vi "Finish.vi"   [LabVIEW 2016]
doc: "This VI is called just before exiting. It is expected to close I/O refnum, save collected data, etc."
uses:
  <vilib>/Rock Robotics/WPI/Utilities/WPI_GetSetVariantRefNum.vi
types:
  T1 = typedef "WPI_MotorControlDeviceRef.ctl" = cluster{"DeviceStatus":errorcluster, "Type":T2, "PWM":cluster{"PWM Channel":T3, "DeadBand":T4}, "CAN":cluster{"Device Number":u8, "SetOutput VI Ref":variant, "GetOutput VI Ref":variant, "Enable VI Ref":variant, "Disable VI Ref":variant, "Data":variant}, "Invert":bool}
  T2 = typedef "WPI_MotorControlType.ctl" = enum16{"PWM", "CAN"}
  T3 = typedef "FPGA_DIOPWMChannel.ctl" = enum8{"PWM 0", "PWM 1", "PWM 2", "PWM 3", "PWM 4", "PWM 5", "PWM 6", "PWM 7", "PWM 8", "PWM 9", "PWM MXP 0", "PWM MXP 1", "PWM MXP 2", "PWM MXP 3", "PWM MXP 4", "PWM MXP 5", "PWM MXP 6", "PWM MXP 7", "PWM MXP 8", "PWM MXP 9", "Invalid"}
  T4 = typedef "WPI_PWMDeadband.ctl" = cluster{"Name":string, "maxPositivePwm":i32, "minPositivePwm":i32, "centerPwm":i32, "maxNegativePwm":i32, "minNegativePwm":i32, "angularRange":u16}
  T5 = typedef "WPI_JoystickDevRef.ctl" = cluster{"Device":T6}
  T6 = typedef "WPI_JoystickDeviceEnum.ctl" = enum16{"USB 0", "USB 1", "USB 2", "USB 3", "USB 4", "USB 5"}
  T7 = typedef "WPI_SolenoidDevRef.ctl" = cluster{"DevStatus":errorcluster, "Pneumatics Control Module":u8, "Forward Solenoid Channel":T8, "Reverse Solenoid Channel":T8}
  T8 = typedef "WPI_SolenoidChannel.ctl" = enum8{"Solenoid 0", "Solenoid 1", "Solenoid 2", "Solenoid 3", "Solenoid 4", "Solenoid 5", "Solenoid 6", "Solenoid 7", "Invalid"}
  T9 = typedef "WPI_CompressorDevRef.ctl" = cluster{"DevStatus":errorcluster, "Pneumatics Control Module":u8}
  T10 = typedef "WPI_EncoderDevRef.ctl" = cluster{"DevStatus":errorcluster, "EncoderIndex":T11, "CounterIndex":T12, "DistancePerCount":dbl, "Decoding Type":T13}
  T11 = typedef "FPGA_EncoderIdx.ctl" = enum8{"Enc 0", "Enc 1", "Enc 2", "Enc 3", "Enc 4", "Enc 5", "Enc 6", "Enc 7", "Invalid"}
  T12 = typedef "FPGA_CounterCtrSystemIndex.ctl" = enum8{"Ctr 0", "Ctr 1", "Ctr 2", "Ctr 3", "Ctr 4", "Ctr 5", "Ctr 6", "Ctr 7", "Invalid"}
  T13 = typedef "WPI_EncoderType.ctl" = enum16{"1x", "2x", "4x"}
  T14 = typedef "WPI_GyroDevRef.ctl" = cluster{"DevStatus":errorcluster, "Analog Channel":T15, "Offset":dbl, "Gain (VoltsPerDegree/Second)":dbl, "Gyro Type":enum16{"Analog", "XRS450"}, "Handle":i32, "SPI Bus":T16, "Device Found":bool, "Sample Rate":dbl, "Calibrate On Open":bool}
  T15 = typedef "FPGA_AIChannel.ctl" = enum8{"AI 0", "AI 1", "AI 2", "AI 3", "AI MXP 0", "AI MXP 1", "AI MXP 2", "AI MXP 3", "Invalid"}
  T16 = typedef "spi_bus.ctl" = enum16{"SPI On-Board, CS0", "SPI On-Board, CS1", "SPI On-Board, CS2", "SPI On-Board, CS3", "SPI MXP", "Invalid"}
  T17 = typedef "WPI_RobotDriveDevRef.ctl" = cluster{"DevStatus":errorcluster, "Motors[]":T1[], "Square Inputs":bool, "Max Output":dbl}
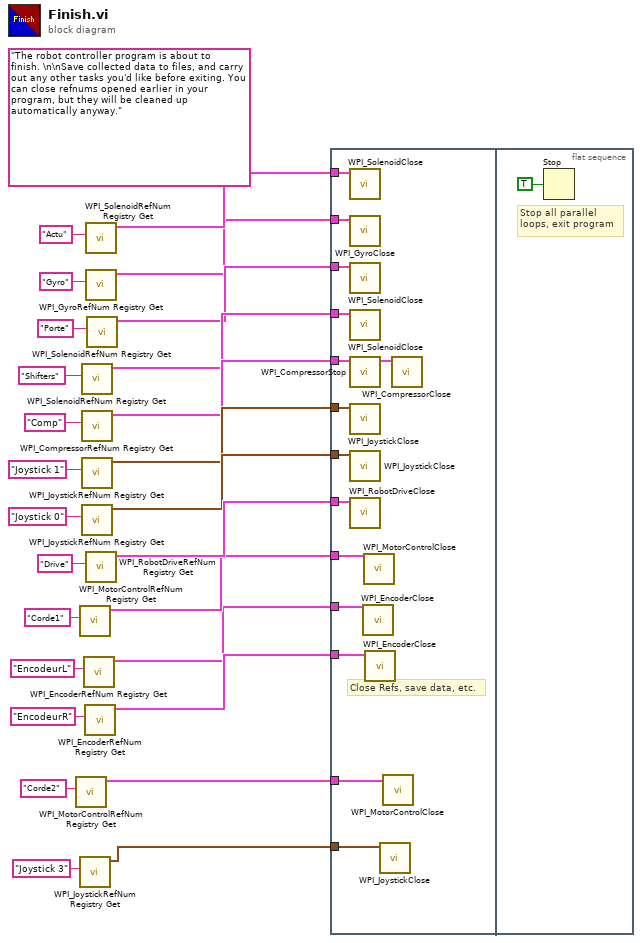
[diagram p0: block diagram]
diagram:
  (unwired) "The robot controller program is about to finish. \n\nSave collected data to files, and carry out any other tasks you'd like before exiting. You can close refnums opened earlier in your program, but they will be cleaned up automatically anyway."
  n1 = call <vilib>:"WPI_MotorControlRefNum Registry Get.vi"("refnum name"="Corde2") -> ("MotorControlDevRef"=w3:T1)  [unwired: 9 in, 1 out]
  n2 = call <vilib>:"WPI_MotorControlRefNum Registry Get.vi"("refnum name"="Corde1") -> ("MotorControlDevRef"=w10:T1)  [unwired: 9 in, 1 out]
  n3 = call <vilib>:"WPI_JoystickRefNum Registry Get.vi"("refnum name"="Joystick 3") -> ("JoystickDevRef"=w4:T5)  [unwired: 9 in, 1 out]
  n4 = call <vilib>:"WPI_SolenoidRefNum Registry Get.vi"("refnum name"="Shifters") -> ("SolenoidDevRef"=w18:T7)  [unwired: 9 in, 1 out]
  n5 = call <vilib>:"WPI_CompressorRefNum Registry Get.vi"("refnum name"="Comp") -> ("CompressorDevRef"=w20:T9)  [unwired: 9 in, 1 out]
  n6 = call <vilib>:"WPI_JoystickRefNum Registry Get.vi"("refnum name"="Joystick 1") -> ("JoystickDevRef"=w21:T5)  [unwired: 1 in, 9 out]
  n7 = call <vilib>:"WPI_JoystickRefNum Registry Get.vi"("refnum name"="Joystick 0") -> ("JoystickDevRef"=w23:T5)  [unwired: 1 in, 9 out]
  n8 = call <vilib>:"WPI_EncoderRefNum Registry Get.vi"("refnum name"="EncodeurL") -> ("EncoderDevRef"=w6:T10)  [unwired: 9 in, 1 out]
  n9 = call <vilib>:"WPI_EncoderRefNum Registry Get.vi"("refnum name"="EncodeurR") -> ("EncoderDevRef"=w8:T10)  [unwired: 9 in, 1 out]
  n10 = call <vilib>:"WPI_SolenoidRefNum Registry Get.vi"("refnum name"="Actu") -> ("SolenoidDevRef"=w16:T7)  [unwired: 9 in, 1 out]
  n11 = call <vilib>:"WPI_GyroRefNum Registry Get.vi"("refnum name"="Gyro") -> ("GyroDevRef"=w12:T14)  [unwired: 9 in, 1 out]
  n12 = call <vilib>:"WPI_RobotDriveRefNum Registry Get.vi"("refnum name"="Drive") -> ("RobotDriveDevRef"=w24:T17)  [unwired: 1 in, 9 out]
  n13 = call <vilib>:"WPI_SolenoidRefNum Registry Get.vi"("refnum name"="Porte") -> ("SolenoidDevRef"=w15:T7)  [unwired: 9 in, 1 out]
  n14 = flat-sequence {
    tunnel: w24 -> [w40]
    tunnel: w23 -> [w39]
    tunnel: w21 -> [w38]
    tunnel: w20 -> [w37]
    tunnel: w18 -> [w35]
    tunnel: w16 -> [w34]
    tunnel: w15 -> [w33]
    tunnel: w12 -> [w32]
    tunnel: w10 -> [w31]
    tunnel: w8 -> [w30]
    tunnel: w6 -> [w29]
    tunnel: w4 -> [w28]
    tunnel: w3 -> [w27]
    frame #0 {
      # "Close Refs, save data, etc."
      n15 = call <vilib>:"WPI_SolenoidClose.vi"("SolenoidDevRef"=w34) -> ()  [unwired: 10 in, 1 out]
      n16 = call <vilib>:"WPI_GyroClose.vi"("GyroDevRef"=w32) -> ()  [unwired: 10 in, 1 out]
      n17 = call <vilib>:"WPI_SolenoidClose.vi"("SolenoidDevRef"=w33) -> ()  [unwired: 10 in, 1 out]
      n18 = call <vilib>:"WPI_SolenoidClose.vi"("SolenoidDevRef"=w35) -> ()  [unwired: 10 in, 1 out]
      n19 = call <vilib>:"WPI_CompressorStop.vi"("CompressorDevRef"=w37) -> ("CompressorDevRef"=w36:T9)  [unwired: 9 in, 1 out]
      n20 = call <vilib>:"WPI_JoystickClose.vi"("JoystickDevRef"=w38) -> ()  [unwired: 11 in]
      n21 = call <vilib>:"WPI_JoystickClose.vi"("JoystickDevRef"=w39) -> ()  [unwired: 11 out]
      n22 = call <vilib>:"WPI_RobotDriveClose.vi"("RobotDriveDevRef"=w40) -> ()  [unwired: 1 in, 10 out]
      n23 = call <vilib>:"WPI_EncoderClose.vi"("EncoderDevRef"=w29) -> ()  [unwired: 10 in, 1 out]
      n24 = call <vilib>:"WPI_MotorControlClose.vi"("MotorControlDevRef"=w31) -> ()  [unwired: 10 in, 1 out]
      n25 = call <vilib>:"WPI_EncoderClose.vi"("EncoderDevRef"=w30) -> ()  [unwired: 10 in, 1 out]
      n26 = call <vilib>:"WPI_JoystickClose.vi"("JoystickDevRef"=w28) -> ()  [unwired: 11 in]
      n27 = call <vilib>:"WPI_MotorControlClose.vi"("MotorControlDevRef"=w27) -> ()  [unwired: 10 in, 1 out]
      n28 = call <vilib>:"WPI_CompressorClose.vi"("CompressorDevRef"=w36) -> ()  [unwired: 10 in, 1 out]
    }
    frame #1 {
      # "Stop all parallel\nloops, exit program"
      n29 = Stop(stop? (T)=TRUE ("Quit")) -> ()
    }
  }
